vi "2D_array_to_string.vi"(1 "2D data array":string[][](array[string]), 2 "Column titles  (separated by tabs)":string, 3 "Array title":string) -> (0 "Output string":string)   [LabVIEW 2020]
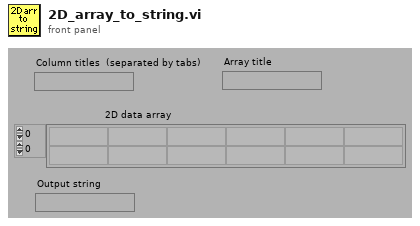
[diagram p1: front panel]
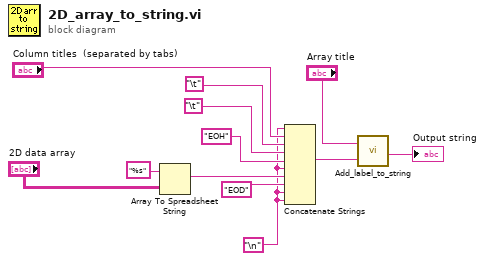
[diagram p0: block diagram]
diagram:
  w1 = "\n"
  n1 = Array To Spreadsheet String(array="2D data array", 3:"%s") -> (spreadsheet string=w11:string)  [unwired: 1 out]
  n2 = Concatenate Strings(w1, "Column titles  (separated by tabs)", "\t", "\t", "EOH", w1, w11, "EOD", w1, w1) -> (w4:string)
  n3 = call "Add_label_to_string.vi"("String to write"=w4, "File Label"="Array title") -> ("Output string"=→"Output string":string)
